vi "Traffic_Lights main.vi"() -> ()   [LabVIEW 2020]
uses:
  #typedef__Semaphore.ctl
  #typedef__States.ctl
  #typedef_timer.ctl
  #typedef__ProgramData.ctl
  #typedef__Semaphores.ctl
  #typedef__LightsTime.ctl
panel:
  in  "stop":bool
  in  "Night Mode End":dbl
  in  "Night Mode Start":dbl
  out "West":T1
  out "North":T1
  out "South":T1
  out "East":T1
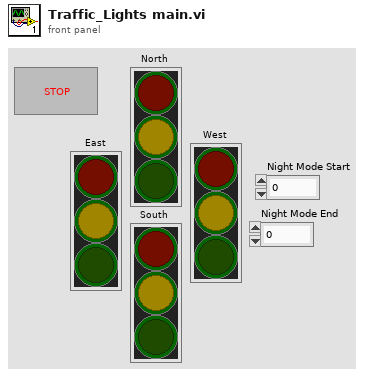
[diagram p1: front panel]
types:
  T1 = typedef "#typedef__Semaphore.ctl" = cluster{"Red":bool, "Yellow":bool, "Green":bool}
  T2 = typedef "#typedef__States.ctl" = enum16{"Initialize", "First_State", "NS_Red", "NS_Yellow", "NS_Green", "EW_Red", "EW_Yellow", "EW_Green", "Night_Yellow", "Night_Empty", "ErrorHandler", "Exit"}
  T3 = typedef "#typedef__ProgramData.ctl" = cluster{"Semaphores":T4, "Lights Time":T5}
  T4 = typedef "#typedef__Semaphores.ctl" = cluster{"East":T1, "South":T1, "North":T1, "West":T1}
  T5 = typedef "#typedef__LightsTime.ctl" = cluster{"Green":dbl, "Yellow":dbl, "Red":dbl, "Night":dbl, "First State":dbl}
  T6 = typedef "#typedef_timer.ctl" = enum16{"Reset", "Run"}
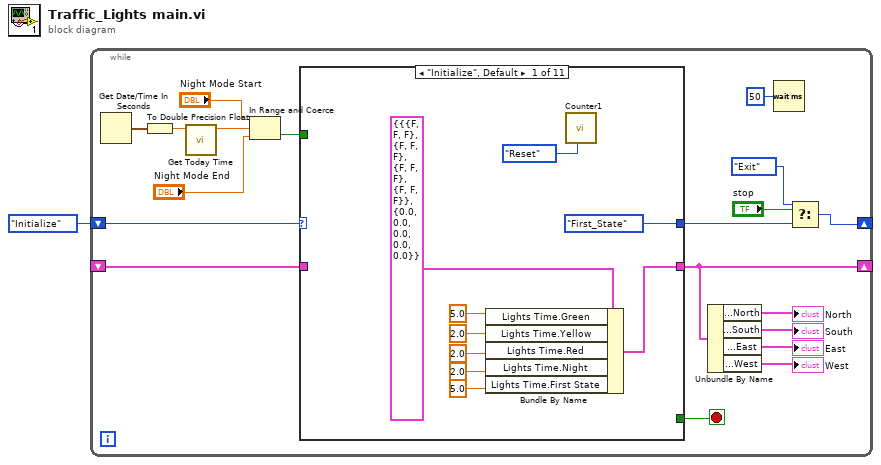
[diagram p0: block diagram]
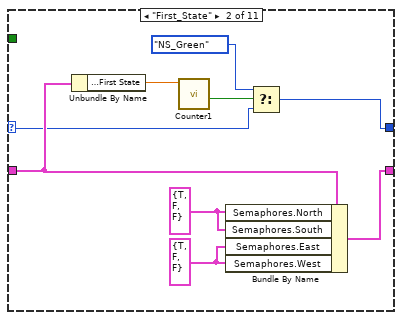
[diagram p2: hidden frame]
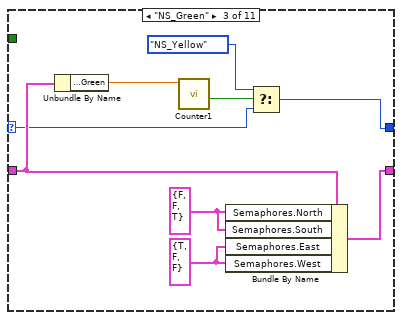
[diagram p3: hidden frame]
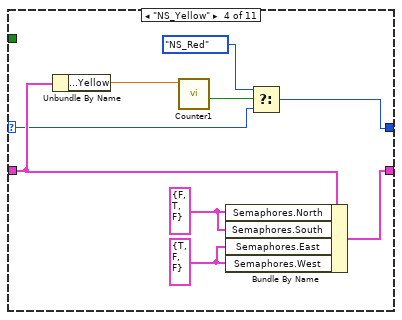
[diagram p4: hidden frame]
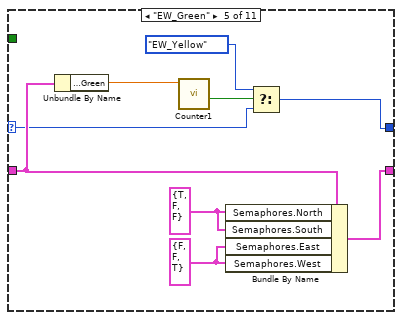
[diagram p5: hidden frame]
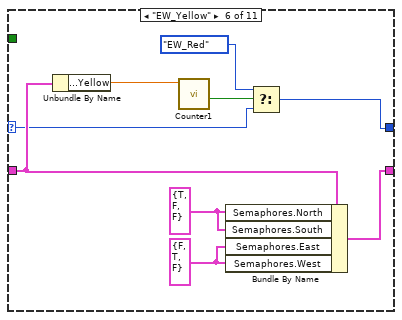
[diagram p6: hidden frame]
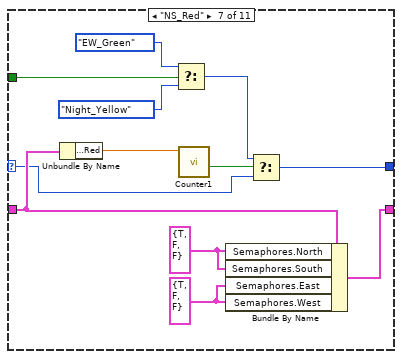
[diagram p7: hidden frame]
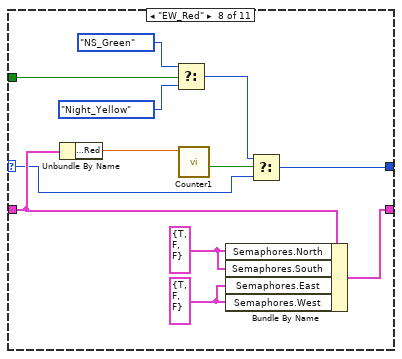
[diagram p8: hidden frame]
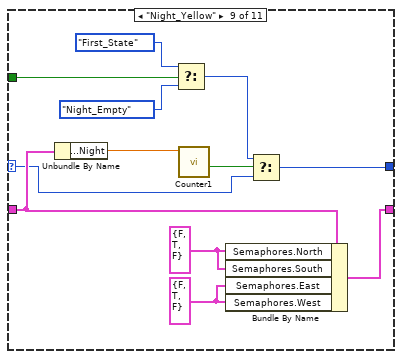
[diagram p9: hidden frame]
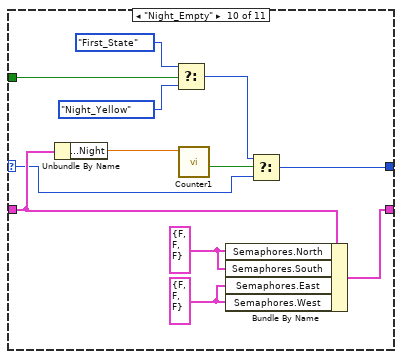
[diagram p10: hidden frame]
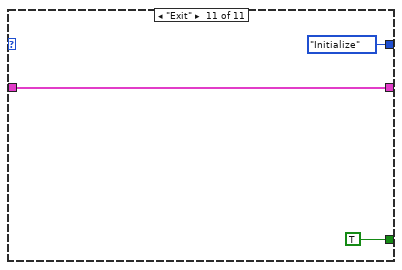
[diagram p11: hidden frame]
diagram:
  n1 = while {
    shift-right: [w4] -> _
    shift-left: #typedef__States."Initialize" ("Enum") -> [w20]
    shift-right: [w19] -> _
    shift-left: _ -> [w14]
    stop <- w7 stop-if-true
    n2 = Get Date/Time In Seconds() -> (seconds since 1Jan1904=w12:timestamp)
    n3 = To Double Precision Float(number=w12) -> (double precision float=w13:dbl)
    n4 = call "Get Today Time.vi"("System Time (s)"=w13) -> ("Today Time"=w11:dbl)  [unwired: 10 in]
    n5 = In Range and Coerce(upper limit="Night Mode Start", x=w11, lower limit="Night Mode End") -> (In Range?=w8:bool)  [unwired: 1 out]
    n6 = case shown="\"Initialize\", Default" w20 {
      selector: w20 -> [_ w31 w40 w49 w58 w67 w80 w92 w104 w116 _]
      tunnel: [#typedef__States."First_State" ("Enum") w30 w39 w48 w57 w66 w79 w91 w103 w115 #typedef__States."Initialize" ("Enum")] -> w5
      tunnel: [w28 w38 w47 w56 w65 w74 w86 w98 w110 w122 w123] -> w19
      tunnel: w14 -> [_ w35 w44 w53 w62 w71 w83 w95 w107 w119 w123]
      tunnel: w8 -> [_ _ _ _ _ _ w78 w90 w102 w114 _]
      tunnel: [_ _ _ _ _ _ _ _ _ _ TRUE] -> w7
      frame "Initialize", Default {
        n7 = Bundle By Name(cluster=T3 {"Semaphores"={"East"={"Red"=FALSE, "Yellow"=FALSE, "Green"=FALSE}, "South"={"Red"=FALSE, "Yellow"=FALSE, "Green"=FALSE}, "North"={"Red"=FALSE, "Yellow"=FALSE, "Green"=FALSE}, "West"={"Red"=FALSE, "Yellow"=FALSE, "Green"=FALSE}}, "Lights Time"={"Green"=0.0, "Yellow"=0.0, "Red"=0.0, "Night"=0.0, "First State"=0.0}} ("Program Data"), "Lights Time.Green"=5.0, "Lights Time.Yellow"=2.0, "Lights Time.Red"=2.0, "Lights Time.Night"=2.0, "Lights Time.First State"=5.0) -> (w28:T3)
        n8 = call "Counter1.vi"("Action (Run)"=#typedef_timer."Reset") -> ()  [unwired: 8 in, 3 out]
      }
      frame "First_State" {
        w36 = T1 {"Red"=TRUE, "Yellow"=FALSE, "Green"=FALSE} ("Semaphore")
        w37 = T1 {"Red"=TRUE, "Yellow"=FALSE, "Green"=FALSE} ("Semaphore")
        n9 = Unbundle By Name(w35) -> ("Lights Time.First State"=w34:dbl)
        n10 = call "Counter1.vi"("Time To Elapse (2s)"=w34) -> ("Time Elapsed?"=w33:bool)  [unwired: 8 in, 2 out]
        n11 = Bundle By Name(cluster=w35, "Semaphores.North"=w36, "Semaphores.South"=w36, "Semaphores.East"=w37, "Semaphores.West"=w37) -> (w38:T3)
        n12 = Select(t=#typedef__States."NS_Green" ("Enum"), s=w33, f=w31) -> (s? t:f=w30:T2)
      }
      frame "NS_Green" {
        w45 = T1 {"Red"=FALSE, "Yellow"=FALSE, "Green"=TRUE} ("Semaphore")
        w46 = T1 {"Red"=TRUE, "Yellow"=FALSE, "Green"=FALSE} ("Semaphore")
        n13 = Unbundle By Name(w44) -> ("Lights Time.Green"=w43:dbl)
        n14 = call "Counter1.vi"("Time To Elapse (2s)"=w43) -> ("Time Elapsed?"=w42:bool)  [unwired: 8 in, 2 out]
        n15 = Bundle By Name(cluster=w44, "Semaphores.North"=w45, "Semaphores.South"=w45, "Semaphores.East"=w46, "Semaphores.West"=w46) -> (w47:T3)
        n16 = Select(t=#typedef__States."NS_Yellow" ("Enum"), s=w42, f=w40) -> (s? t:f=w39:T2)
      }
      frame "NS_Yellow" {
        w54 = T1 {"Red"=FALSE, "Yellow"=TRUE, "Green"=FALSE} ("Semaphore")
        w55 = T1 {"Red"=TRUE, "Yellow"=FALSE, "Green"=FALSE} ("Semaphore")
        n17 = Unbundle By Name(w53) -> ("Lights Time.Yellow"=w52:dbl)
        n18 = call "Counter1.vi"("Time To Elapse (2s)"=w52) -> ("Time Elapsed?"=w51:bool)  [unwired: 8 in, 2 out]
        n19 = Bundle By Name(cluster=w53, "Semaphores.North"=w54, "Semaphores.South"=w54, "Semaphores.East"=w55, "Semaphores.West"=w55) -> (w56:T3)
        n20 = Select(t=#typedef__States."NS_Red" ("Enum"), s=w51, f=w49) -> (s? t:f=w48:T2)
      }
      frame "EW_Green" {
        w63 = T1 {"Red"=TRUE, "Yellow"=FALSE, "Green"=FALSE} ("Semaphore")
        w64 = T1 {"Red"=FALSE, "Yellow"=FALSE, "Green"=TRUE} ("Semaphore")
        n21 = Unbundle By Name(w62) -> ("Lights Time.Green"=w61:dbl)
        n22 = call "Counter1.vi"("Time To Elapse (2s)"=w61) -> ("Time Elapsed?"=w60:bool)  [unwired: 8 in, 2 out]
        n23 = Bundle By Name(cluster=w62, "Semaphores.North"=w63, "Semaphores.South"=w63, "Semaphores.East"=w64, "Semaphores.West"=w64) -> (w65:T3)
        n24 = Select(t=#typedef__States."EW_Yellow" ("Enum"), s=w60, f=w58) -> (s? t:f=w57:T2)
      }
      frame "EW_Yellow" {
        w72 = T1 {"Red"=TRUE, "Yellow"=FALSE, "Green"=FALSE} ("Semaphore")
        w73 = T1 {"Red"=FALSE, "Yellow"=TRUE, "Green"=FALSE} ("Semaphore")
        n25 = Unbundle By Name(w71) -> ("Lights Time.Yellow"=w70:dbl)
        n26 = call "Counter1.vi"("Time To Elapse (2s)"=w70) -> ("Time Elapsed?"=w69:bool)  [unwired: 8 in, 2 out]
        n27 = Bundle By Name(cluster=w71, "Semaphores.North"=w72, "Semaphores.South"=w72, "Semaphores.East"=w73, "Semaphores.West"=w73) -> (w74:T3)
        n28 = Select(t=#typedef__States."EW_Red" ("Enum"), s=w69, f=w67) -> (s? t:f=w66:T2)
      }
      frame "NS_Red" {
        w84 = T1 {"Red"=TRUE, "Yellow"=FALSE, "Green"=FALSE} ("Semaphore")
        w85 = T1 {"Red"=TRUE, "Yellow"=FALSE, "Green"=FALSE} ("Semaphore")
        n29 = Unbundle By Name(w83) -> ("Lights Time.Red"=w82:dbl)
        n30 = Select(t=#typedef__States."EW_Green" ("Enum"), s=w78, f=#typedef__States."Night_Yellow") -> (s? t:f=w75:T2)
        n31 = call "Counter1.vi"("Time To Elapse (2s)"=w82) -> ("Time Elapsed?"=w81:bool)  [unwired: 8 in, 2 out]
        n32 = Bundle By Name(cluster=w83, "Semaphores.North"=w84, "Semaphores.South"=w84, "Semaphores.East"=w85, "Semaphores.West"=w85) -> (w86:T3)
        n33 = Select(t=w75, s=w81, f=w80) -> (s? t:f=w79:T2)
      }
      frame "EW_Red" {
        w96 = T1 {"Red"=TRUE, "Yellow"=FALSE, "Green"=FALSE} ("Semaphore")
        w97 = T1 {"Red"=TRUE, "Yellow"=FALSE, "Green"=FALSE} ("Semaphore")
        n34 = Unbundle By Name(w95) -> ("Lights Time.Red"=w94:dbl)
        n35 = Select(t=#typedef__States."NS_Green" ("Enum"), s=w90, f=#typedef__States."Night_Yellow") -> (s? t:f=w87:T2)
        n36 = call "Counter1.vi"("Time To Elapse (2s)"=w94) -> ("Time Elapsed?"=w93:bool)  [unwired: 8 in, 2 out]
        n37 = Bundle By Name(cluster=w95, "Semaphores.North"=w96, "Semaphores.South"=w96, "Semaphores.East"=w97, "Semaphores.West"=w97) -> (w98:T3)
        n38 = Select(t=w87, s=w93, f=w92) -> (s? t:f=w91:T2)
      }
      frame "Night_Yellow" {
        w108 = T1 {"Red"=FALSE, "Yellow"=TRUE, "Green"=FALSE} ("Semaphore")
        w109 = T1 {"Red"=FALSE, "Yellow"=TRUE, "Green"=FALSE} ("Semaphore")
        n39 = Unbundle By Name(w107) -> ("Lights Time.Night"=w106:dbl)
        n40 = Select(t=#typedef__States."First_State" ("Enum"), s=w102, f=#typedef__States."Night_Empty") -> (s? t:f=w99:T2)
        n41 = call "Counter1.vi"("Time To Elapse (2s)"=w106) -> ("Time Elapsed?"=w105:bool)  [unwired: 8 in, 2 out]
        n42 = Bundle By Name(cluster=w107, "Semaphores.North"=w108, "Semaphores.South"=w108, "Semaphores.East"=w109, "Semaphores.West"=w109) -> (w110:T3)
        n43 = Select(t=w99, s=w105, f=w104) -> (s? t:f=w103:T2)
      }
      frame "Night_Empty" {
        w120 = T1 {"Red"=FALSE, "Yellow"=FALSE, "Green"=FALSE} ("Semaphore")
        w121 = T1 {"Red"=FALSE, "Yellow"=FALSE, "Green"=FALSE} ("Semaphore")
        n44 = Unbundle By Name(w119) -> ("Lights Time.Night"=w118:dbl)
        n45 = Select(t=#typedef__States."First_State" ("Enum"), s=w114, f=#typedef__States."Night_Yellow") -> (s? t:f=w111:T2)
        n46 = call "Counter1.vi"("Time To Elapse (2s)"=w118) -> ("Time Elapsed?"=w117:bool)  [unwired: 8 in, 2 out]
        n47 = Bundle By Name(cluster=w119, "Semaphores.North"=w120, "Semaphores.South"=w120, "Semaphores.East"=w121, "Semaphores.West"=w121) -> (w122:T3)
        n48 = Select(t=w111, s=w117, f=w116) -> (s? t:f=w115:T2)
      }
      frame "Exit" {
      }
    }
    n49 = Unbundle By Name(w19) -> ("Semaphores.North"=→"North":T1, "Semaphores.South"=→"South":T1, "Semaphores.East"=→"East":T1, "Semaphores.West"=→"West":T1)
    n50 = Wait (ms)(milliseconds to wait=u32 50) -> ()  [unwired: 1 out]
    n51 = Select(t=#typedef__States."Exit" ("Enum"), s="stop", f=w5) -> (s? t:f=w4:T2)
  }
